vi "rad_Verify Image Compatibility.vi"(6 "Require Identical Chassis?":bool, 8 "error in (no error)":errorcluster, 10 "Target address":T4={"Hostname"="", "Serial number"="", "Product name"="", "Product code"=0, "System status"="", "Credential type"=enum."None/Unlocked", "User added?"=FALSE, "Primary NIC"={"MAC address"="", "IP Address Request Mode"=2, "IP address"="", "Subnet mask"="", "Gateway"="", "DNS server"=""}} {"Primary NIC"."IP Address Request Mode" items=["Static"=1, "DHCP/Link-Local"=2, "Link-Local Only"=4, "DHCP Only"=8]}, 11 "AppImage Properties":T1) -> (0 "error out":errorcluster, 3 "Compatible?":bool, 5 "Status message":string)   [LabVIEW 2020]
uses:
  Targets/TypeDefs/rad_Target Information.ctl
  Targets/TypeDefs/rad_Target Network Settings.ctl
  TypeDefs/rad_Application Image Properties.ctl
  TypeDefs/rad_FPGA Properties.ctl
  TypeDefs/rad_FPGA Flash Properties.ctl
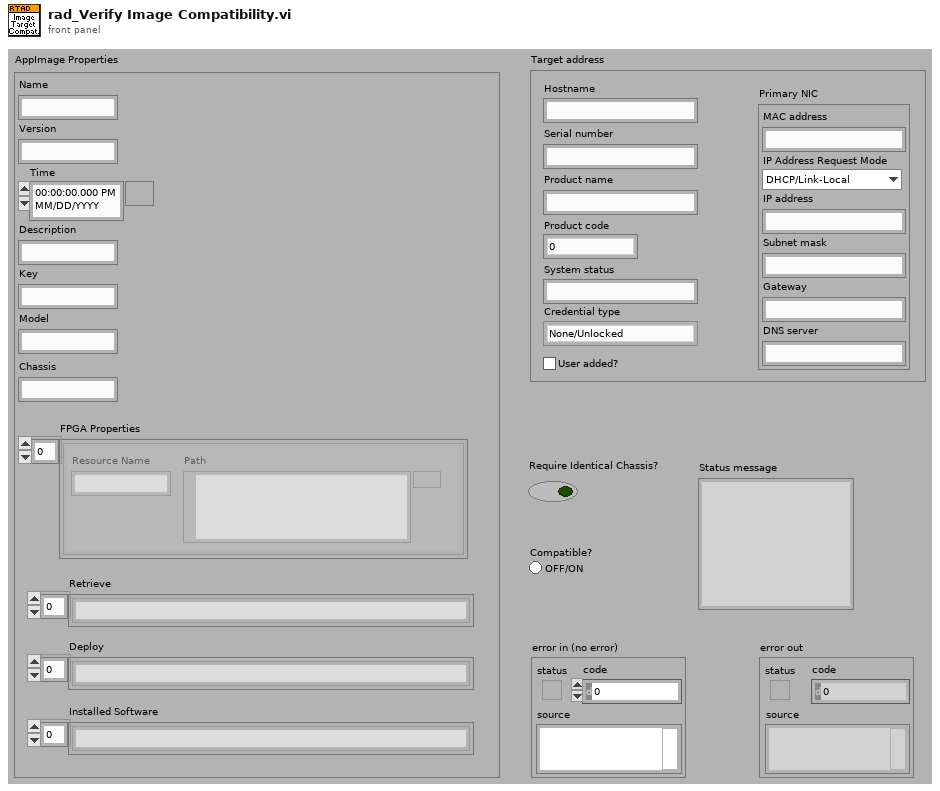
[diagram p1: front panel]
types:
  T1 = typedef "rad_Application Image Properties.ctl" = cluster{"Name":string, "Version":string, "Time":timestamp, "Description":string, "Key":string, "Chassis":string, "FPGA Properties":T2, "Model":string, "Retrieve":string[], "Deploy":string[], "Installed Software":string[]}
  T2 = typedef "rad_FPGA Properties.ctl" = T3[]
  T3 = typedef "rad_FPGA Flash Properties.ctl" = cluster{"Resource Name":string, "Path":path}
  T4 = typedef "rad_Target Information.ctl" = cluster{"Hostname":string, "Serial number":string, "Product name":string, "Product code":i32, "System status":string, "Credential type":enum16{"None/Unlocked", "FTP Password", "NIAuth Credentials"}, "User added?":bool, "Primary NIC":T5}
  T5 = typedef "rad_Target Network Settings.ctl" = cluster{"MAC address":string, "IP Address Request Mode":i32, "IP address":string, "Subnet mask":string, "Gateway":string, "DNS server":string}
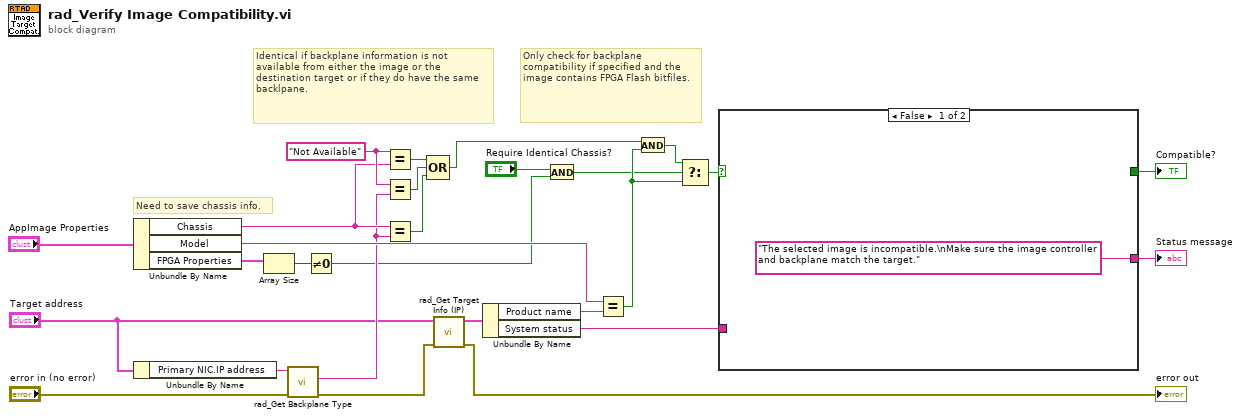
[diagram p0: block diagram]
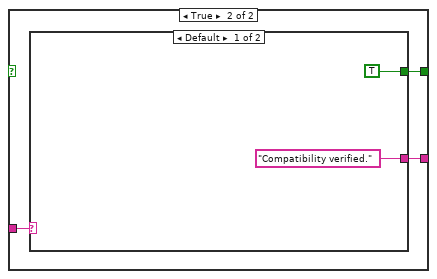
[diagram p2: hidden frame]
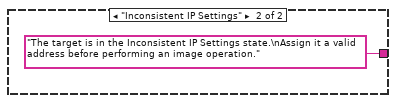
[diagram p3: hidden frame]
diagram:
  w23 = "Not Available"
  # "Only check for backplane compatibility if specified and the image contains FPGA Flash bitfiles."
  # "Identical if backplane information is not available from either the image or the destination target or if they do have the same backlpane."
  # "Need to save chassis info."
  n1 = Unbundle By Name("AppImage Properties") -> ("Chassis"=w22:string, "Model"=w24:string, "FPGA Properties"=w14:T2)
  n2 = Unbundle By Name("Target address") -> ("Primary NIC.IP address"=w3:string)
  n3 = Array Size(array=w14) -> (size(s)=w13:i32)
  n4 = call "rad_Get Backplane Type.vi"("error in (no error)"="error in (no error)", "Controller IP"=w3) -> ("error out"=w2:errorcluster, "Backplane Type"=w17:string)  [unwired: 7 in, 1 out]
  n5 = Not Equal To 0?(x=w13) -> (x != 0?=w11:bool)
  n6 = Equal?(x=w23, y=w22) -> (x = y?=w21:bool)
  n7 = Equal?(x=w23, y=w17) -> (x = y?=w20:bool)
  n8 = Equal?(x=w22, y=w17) -> (x = y?=w19:bool)
  n9 = Compound Arithmetic op=OR(w21, w20, w19) -> (w18:bool)
  n10 = call "rad_Get Target Info (IP).vi"("error in (no error)"=w2, "Target settings in"="Target address") -> ("error out"=→"error out":errorcluster, "Target settings out"=w15:T4)  [unwired: 8 in]
  n11 = Unbundle By Name(w15) -> ("Product name"=w27:string, "System status"=w4:string)
  n12 = And(x="Require Identical Chassis?", y=w11) -> (x .and. y?=w10:bool)
  n13 = Equal?(x=w24, y=w27) -> (x = y?=w26:bool)
  n14 = And(x=w18, y=w26) -> (x .and. y?=w25:bool)
  n15 = Select(t=w25, s=w10, f=w26) -> (s? t:f=w7:bool)
  n16 = case shown="False" w7 {
    tunnel: [_ w30] -> w6
    tunnel: ["The selected image is incompatible.\nMake sure the image controller and backplane match the target." w29] -> w5
    tunnel: w4 -> [_ w31]
    frame False {
    }
    frame True {
      n17 = case shown="Default" w31 {
        tunnel: [TRUE _] -> w30
        tunnel: ["Compatibility verified." ("f") "The target is in the Inconsistent IP Settings state.\nAssign it a valid address before performing an image operation."] -> w29
        frame Default {
        }
        frame "Inconsistent IP Settings" {
        }
      }
    }
  }
  "Compatible?" <- w6
  "Status message" <- w5
